vi "WPI_AccumulatorGetConfiguration.vi"(8 "error in (no error)":errorcluster, 11 "AIDeviceRef":T1={"DevStatus"={"status"=FALSE, "code"=0, "source"=""}, "Analog Channel"=enum."AI 1"}) -> (0 "error out":errorcluster, 1 "Initial Value":dbl, 2 "Center":dbl, 3 "AIDeviceRef":T1={"DevStatus"={"status"=FALSE, "code"=0, "source"=""}, "Analog Channel"=enum."AI 1"}, 4 "Deadband":dbl)   [LabVIEW 2017]
doc: "Returns the center value, initial value, and deadband of the accumulator on the FPGA on the roboRIO device. The FPGA subtracts the center value from the value of each element before adding the value of the element to the cumulative value of the accumulator. You can use the center value and initial value to account for offset in devices, such as gyros and accelerometers, when integrating signals from these devices. The accumulator does not accumulate a value if the difference between the center value and the current value is less than the deadband.\n\nThis software is licensed. Open the labview\\readme\\WPI Robotics Library Open Source License.txt file for more information."
uses:
  <vilib>/Rock Robotics/WPI/AnalogChannel/WPI_AnalogChannelDevRef.ctl
  <vilib>/Rock Robotics/SystemInterfaces/AI/FPGA_AIChannel.ctl
  <vilib>/Rock Robotics/SystemInterfaces/System/FPGA_SystemGet.vi
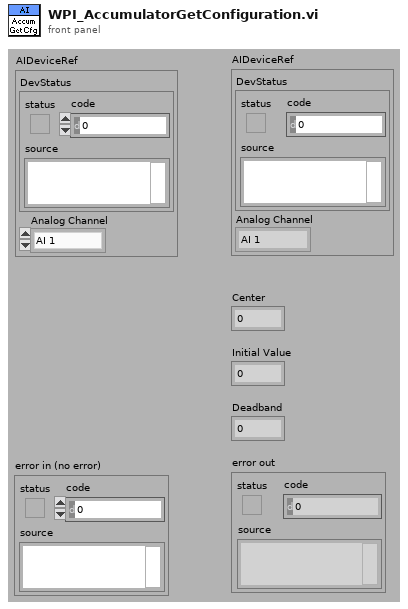
[diagram p1: front panel]
types:
  T1 = typedef "WPI_AnalogChannelDevRef.ctl" = cluster{"DevStatus":errorcluster, "Analog Channel":T2}
  T2 = typedef "FPGA_AIChannel.ctl" = enum8{"AI 0", "AI 1", "AI 2", "AI 3", "AI MXP 0", "AI MXP 1", "AI MXP 2", "AI MXP 3", "Invalid"}
  T3 = typedef "FPGA_AIDevRef.ctl" = cluster{"DevStatus":errorcluster}
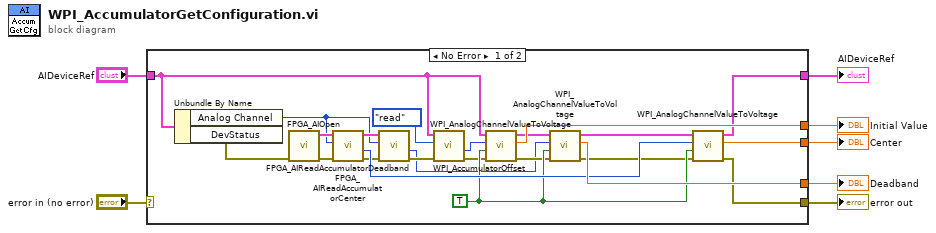
[diagram p0: block diagram]
diagram:
  n1 = case shown="No Error" "error in (no error)" {
    selector: "error in (no error)" -> [_ w31]
    tunnel: [w17 w32] -> w7
    tunnel: "AIDeviceRef" -> [w28 w32]
    tunnel: [w16 w31] -> w4
    tunnel: [w18 _] -> w3
    tunnel: [w22 _] -> w2
    tunnel: [w20 _] -> w1
    frame No Error {
      w15 = TRUE ("Averaged")
      n2 = Unbundle By Name(w28) -> ("Analog Channel"=w24:T2, "DevStatus"=w30:errorcluster)
      n3 = call <vilib>:"FPGA_AIOpen.vi"("error in (no error)"=w30) -> ("error out"=w13:errorcluster, "AI Reference out"=w29:T3)  [unwired: 2 in, 7 out]
      n4 = call <vilib>:"FPGA_AIReadAccumulatorCenter.vi"("error in (no error)"=w13, "Channel"=w24, "AI Reference in"=w29) -> ("error out"=w12:errorcluster, "Center"=w19:i32, "AI Reference out"=w26:T3)  [unwired: 6 out]
      n5 = call <vilib>:"FPGA_AIReadAccumulatorDeadband.vi"("error in (no error)"=w12, "Channel"=w24, "AI Reference in"=w26) -> ("error out"=w25:errorcluster, "Deadband"=w8:i32)  [unwired: 7 out]
      n6 = call <vilib>:"WPI_AccumulatorOffset.vi"("error in (no error)"=w25, "Action"=enum16{"read", "write"}."read" ("what do"), "AIDeviceRef"=w28) -> ("error out"=w14:errorcluster, "Offset Out"=w23:i32)  [unwired: 1 in, 6 out]
      n7 = call <vilib>:"WPI_AnalogChannelValueToVoltage.vi"("error in (no error)"=w14, "Averaged"=w15, "Value"=w23, "AIDeviceRef"=w28) -> ("error out"=w11:errorcluster, "Voltage"=w22:dbl, "AIDeviceRef"=w21:T1)  [unwired: 1 in, 4 out]
      n8 = call <vilib>:"WPI_AnalogChannelValueToVoltage.vi"("error in (no error)"=w11, "Averaged"=w15, "Value"=w8, "AIDeviceRef"=w21) -> ("error out"=w10:errorcluster, "Voltage"=w20:dbl, "AIDeviceRef"=w9:T1)  [unwired: 1 in, 4 out]
      n9 = call <vilib>:"WPI_AnalogChannelValueToVoltage.vi"("error in (no error)"=w10, "Averaged"=w15, "Value"=w19, "AIDeviceRef"=w9) -> ("error out"=w16:errorcluster, "Voltage"=w18:dbl, "AIDeviceRef"=w17:T1)  [unwired: 1 in, 4 out]
    }
    frame Error {
    }
  }
  "AIDeviceRef" <- w7
  "Center" <- w3
  "error out" <- w4
  "Initial Value" <- w2
  "Deadband" <- w1
